vi "decode access token response.vi"(8 "error in (no error)":errorcluster, 9 "Response":string, 10 "Header":string, 11 "Oauth2 in":refnum<class "Oauth2.lvclass">) -> (0 "error out":errorcluster, 3 "Oauth2":refnum<class "Oauth2.lvclass">)   [LabVIEW 2017, in "Oauth2.lvclass"]
uses:
  Oauth2.lvclass
  OAuthToken/OAuth2 Token Element -- enum.ctl
  OAuthToken/OAuthAccessToken.lvclass
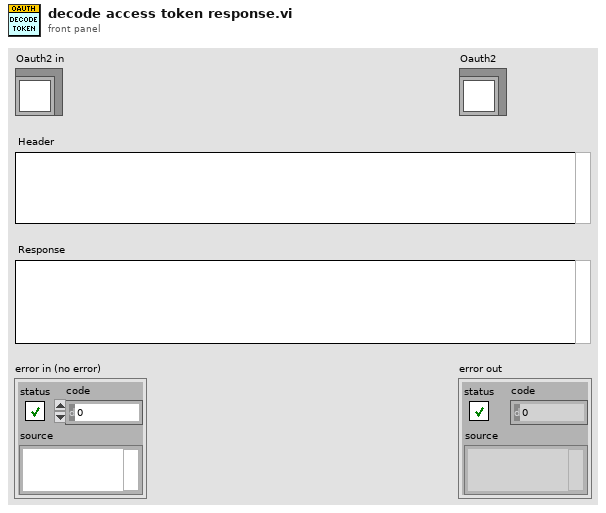
[diagram p1: front panel]
types:
  T1 = typedef "OAuthAccessToken.lvclass/OAuth2 Token Element -- enum.ctl" = enum16{"client_id", "client_secret", "response_type", "scope", "redirect_uri", "error", "error_description", "error_uri", "grant_type", "code", "access_token", "token_type", "expires_in", "username", "password", "refresh_token", "code_challenge", "code_challenge_method", "reverse_proxy_uri", "endpoint element", "prompt", "access_type", "id_token"}
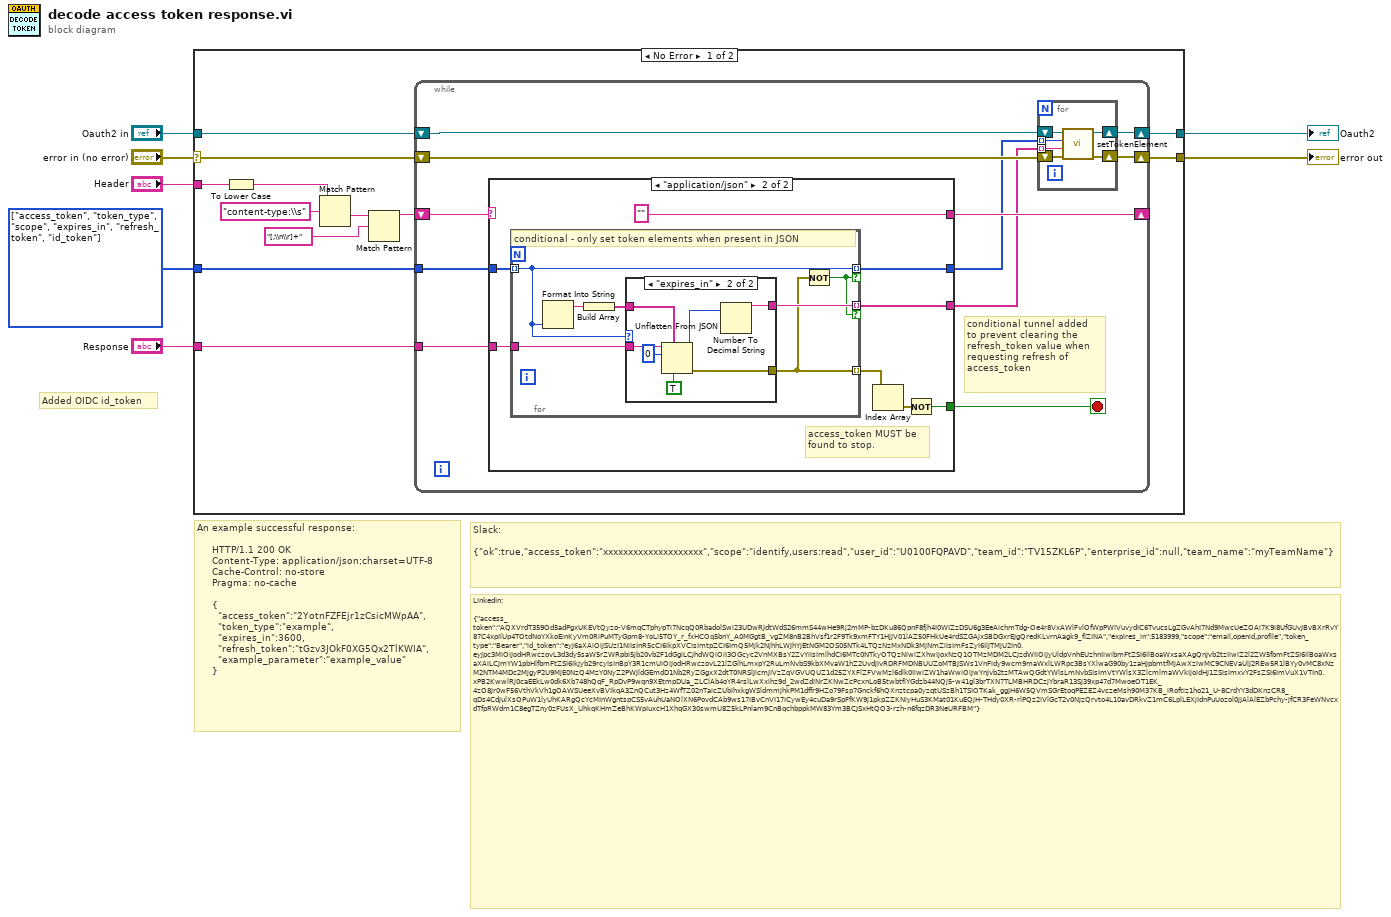
[diagram p0: block diagram]
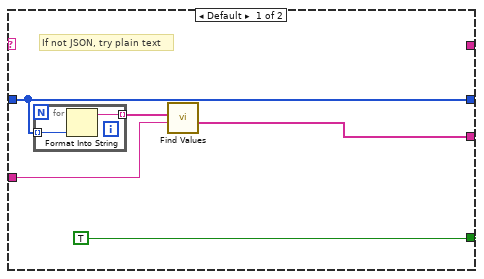
[diagram p2: hidden frame]
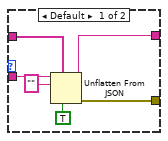
[diagram p3: hidden frame]
diagram:
  w1 = T1[] [enum."access_token", enum."token_type", enum."scope", enum."expires_in", enum."refresh_token", enum."id_token"] items=["client_id", "client_secret", "response_type", "scope", "redirect_uri", "error", "error_description", "error_uri", "grant_type", "code", "access_token", "token_type", "expires_in", "username", "password", "refresh_token", "code_challenge", "code_challenge_method", "reverse_proxy_uri", "endpoint element", "prompt", "access_type", "id_token"]
  # "Added OIDC id_token"
  # "LinkedIn:\n\n{\"access_token\":\"AQXVrdT359Od5adPgxUKEVtQyzo-V6mqCTphypTi7NcqQ0RbadolSwi23UDwRJdtWdS26mmS44wHe9Rj2mMP-bzDKu86QpnF8fjh4I0WIZzDSU6g3EeAichmTdg-Oe4r8VxAWlFvlOfWpPWIVuvydIC6TvucsLgZGvAhI7Nd9MwcUeZOAi7K9i8UfGUvJBvBXrRvY87C4xpIlUp4TOtdNoYXkoEinKyVm0RiPuMTyGpm8-YoLi5TOY_r_fxHCOq5bnY_A0MGgtB_vgZM8nB2BhVsf1r2F9Tk9xmFTY1HjJV01lAZ50FHkUe4rdSZGAjxSBDGxrEJgQredKLvrnAagk9_fIZINA\",\"expires_in\":5183999,\"scope\":\"email,openid,profile\",\"token_type\":\"Bearer\",\"id_token\":\"eyJ6aXAiOiJSUzI1NiIsInR5cCI6IkpXVCIsImtpZCI6ImQ5Mjk2NjhhLWJhYjEtNGM2OS05NTk4LTQzNzMxNDk3MjNmZiIsImFsZyI6IlJTMjU2In0.eyJpc3MiOiJodHRwczovL3d3dy5saW5rZWRpbi5jb20vb2F1dGgiLCJhdWQiOiI3OGcyc2VnMXBsY2ZvYiIsImlhdCI6MTc0NTkyOTQzNiwiZXhwIjoxNzQ1OTMzMDM2LCJzdWIiOiJyUldpVnhEUzhnIiwibmFtZSI6IlBoaWxsaXAgQnJvb2tzIiwiZ2l2ZW5fbmFtZSI6IlBoaWxsaXAiLCJmYW1pbHlfbmFtZSI6IkJyb29rcyIsInBpY3R1cmUiOiJodHRwczovL21lZGlhLmxpY2RuLmNvbS9kbXMvaW1hZ2UvdjIvRDRFMDNBUUZoMTBJSWs1VnFidy9wcm9maWxlLWRpc3BsYXlwaG90by1zaHJpbmtfMjAwXzIwMC9CNEVaUlJ2REw5R1lBYy0vMC8xNzM2NTM4MDc2MjgyP2U9MjE0NzQ4MzY0NyZ2PWJldGEmdD1Nb2RyZGgxX2dtT0NRSlJicmJIVzZqVGVUQUZ1d25ZYXFlZFVwMzl6dlk0IiwiZW1haWwiOiJwYnJvb2tzMTAwQGdtYWlsLmNvbSIsImVtYWlsX3ZlcmlmaWVkIjoidHJ1ZSIsImxvY2FsZSI6ImVuX1VTIn0.xPB2KwwlRj0caEEkLw0dk6Xb748hQqF_RpDvP9wqn9XEtmpDUa_ZLClAb4oYR4rslLwXxihz9d_2wdZdiNrZKNwZcPcxnLoB5twbtflYGdzb44NQj5-w41gl3brTXN7TLMBHRDCzjYbraR13SJ39xp47d7MwoeOT1EK_4zO8Jr0wF56VthVkVh1gOAWSUeeXvBVIkqA3ZnQCut3Hz4WfTZ02nTaicZUbIhxkgWSldmmjhkPM1dffr9HZo79Fsp7Gnckf6hQXnztcpa0yzqtUSzBh1TSIOTKak_ggJH6W5QVmSGrEtoqPEZEZ4vczeMsh90M37KB_iRoftiz1ho21_U-8CrdYY3dDKnzCR8_qDs4CdJulXsOPuW1lyUhKARgQcYcMInWgntspCS5vAuhUaNOlXN6PovdCAb9ws17iBvCnVI17iCywEy4cuDa9rSpFfKW9j1pkpZZKNiyHuS3KMat01KuEQjH-THdy0XR-rlPQz2iVlGcT2v0NjzQrvto4L10avDRkvZ1mC6LplLEXjIdnPuUozol0jJAlAlEZbPchy-jfCR3FeWNvcxdTfpRWdm1C8egTZny0zFUsX_UhkqKHmZeBhKWpIuxcH1XhqGX30swmU8Z5kLPnlam9CnBqchbppkMW83Ym3BCJSxHtQO3-rzh-n6fqzDR3NeURFBM\"}"
  # "Slack:\n\n{\"ok\":true,\"access_token\":\"xxxxxxxxxxxxxxxxxxxx\",\"scope\":\"identify,users:read\",\"user_id\":\"U0100FQPAVD\",\"team_id\":\"TV15ZKL6P\",\"enterprise_id\":null,\"team_name\":\"myTeamName\"}"
  # "An example successful response:\n\n     HTTP/1.1 200 OK\n     Content-Type: application/json;charset=UTF-8\n     Cache-Control: no-store\n     Pragma: no-cache\n\n     {\n       \"access_token\":\"2YotnFZFEjr1zCsicMWpAA\",\n       \"token_type\":\"example\",\n       \"expires_in\":3600,\n       \"refresh_token\":\"tGzv3JOkF0XG5Qx2TlKWIA\",\n       \"example_parameter\":\"example_value\"\n     }"
  n1 = case shown="No Error" "error in (no error)" {
    selector: "error in (no error)" -> [w8 w73]
    tunnel: [w17 w73] -> w6
    tunnel: [w18 w72] -> w4
    tunnel: "Oauth2 in" -> [w9 w72]
    tunnel: "Response" -> [w19 _]
    tunnel: "Header" -> [w16 _]
    tunnel: w1 -> [w11 _]
    frame No Error {
      n2 = To Lower Case(string=w16) -> (all lower case string=w10:string)
      n3 = Match Pattern(string=w10, regular expression="content-type:\\s") -> (after substring=w14:string)  [unwired: 1 in, 3 out]
      n4 = Match Pattern(string=w14, regular expression="[;\\n\\r]+") -> (before substring=w12:string)  [unwired: 1 in, 3 out]
      n5 = while {
        tunnel: w19 -> [w30]
        shift-right: [w25] -> w18
        shift-left: w9 -> [w23]
        shift-right: [w24] -> w17
        shift-left: w8 -> [w22]
        shift-right: [w27] -> _
        shift-left: w12 -> [w28]
        tunnel: w11 -> [w26]
        stop <- w29 stop-if-true
        # "conditional tunnel added\nto prevent clearing the \nrefresh_token value when \nrequesting refresh of \naccess_token"
        n6 = case shown="\"application/json\"" w28 {
          tunnel: w30 -> [w38 w51]
          tunnel: [TRUE w48] -> w29
          tunnel: [_ "" ("regular expression")] -> w27
          tunnel: w26 -> [w40 w46]
          tunnel: [w40 w45] -> w21
          tunnel: [w37 w44] -> w20
          frame Default {
            # "If not JSON, try plain text"
            n7 = for {
              tunnel: w40 -> [w43] mode=indexing
              tunnel: [w42] -> w39 mode=indexing
              n8 = Format Into String(w43) -> (resulting string=w42:string)  [unwired: 3 in, 1 out]
            }
            n9 = call "Find Values.vi"("Response string"=w38, "keys"=w39) -> ("values"=w37:string[])  [unwired: 8 in, 1 out]
          }
          frame "application/json" {
            # "access_token MUST be\nfound to stop."
            n10 = for {
              tunnel: w51 -> [w58]
              tunnel: [w53] -> w50 mode=indexing
              tunnel: w46 -> [w54] mode=indexing
              tunnel: [w54] -> w45 mode=indexing if=w52
              tunnel: [w56] -> w44 mode=indexing if=w52
              # "conditional - only set token elements when present in JSON"
              n11 = Format Into String(w54) -> (resulting string=w57:string)  [unwired: 3 in, 1 out]
              n12 = Build Array(w57) -> (w55:string[])
              n13 = case shown="\"expires_in\"" w54 {
                tunnel: w58 -> [w64 w71]
                tunnel: [w63 w70] -> w53
                tunnel: [w61 w66] -> w56
                tunnel: w55 -> [w60 w68]
                frame Default {
                  n14 = Unflatten From JSON(path=w60, JSON string=w64, type and defaults="", default null elements? (F)=TRUE) -> (value=w61:string, error out=w63:errorcluster)  [unwired: 3 in]
                }
                frame "expires_in" {
                  n15 = Unflatten From JSON(path=w68, JSON string=w71, type and defaults=u32 0, default null elements? (F)=TRUE) -> (value=w65:u32, error out=w70:errorcluster)  [unwired: 3 in]
                  n16 = Number To Decimal String(number=w65) -> (decimal integer string=w66:string)  [unwired: 1 in]
                }
              }
              n17 = Not(x=w53) -> (.not. x?=w52:bool)
            }
            n18 = Index Array(array=w50) -> (element=w49:errorcluster)  [unwired: 1 in]
            n19 = Not(x=w49) -> (.not. x?=w48:bool)
          }
        }
        n20 = for {
          shift-right: [w35] -> w25
          shift-left: w23 -> [w36]
          shift-right: [w33] -> w24
          shift-left: w22 -> [w34]
          tunnel: w21 -> [w32] mode=indexing
          tunnel: w20 -> [w31] mode=indexing
          n21 = call "setTokenElement.vi"("error in (no error)"=w34, "Value"=w31, "Token element"=w32, "Oauth2 in"=w36) -> ("error out"=w33:errorcluster, "Oauth2 out"=w35:refnum<class "Oauth2.lvclass">)  [unwired: 6 in]
        }
      }
    }
    frame Error {
    }
  }
  "error out" <- w6
  "Oauth2" <- w4
